vi "Set Slaves in HWI.vi"(8 "error in (no error)":errorcluster, 10 "Slave Info":T1, 11 "Pulseblaster in":refnum<class "Pulseblaster.lvclass">) -> (0 "error out":errorcluster, 3 "Pulseblaster out":refnum<class "Pulseblaster.lvclass">)   [LabVIEW 2013, in "Pulseblaster.lvclass"]
uses:
  Pulseblaster.lvclass
  TypeDefs/SlaveInfo.ctl
  TypeDefs/RampInfo.ctl
  Pulseblaster.lvclass/Pulseblaster.ctl
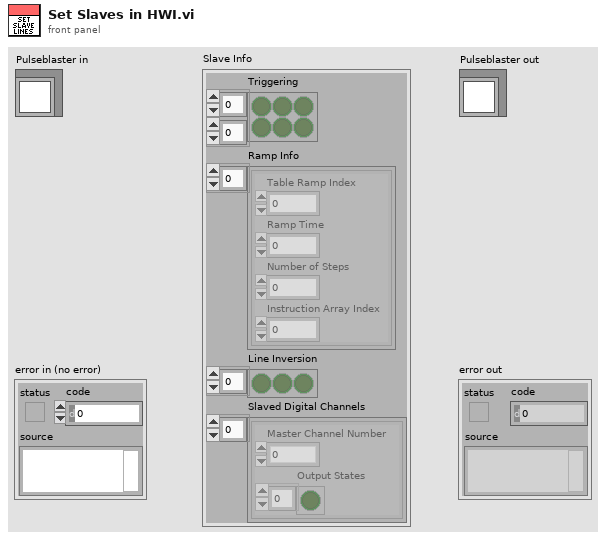
[diagram p1: front panel]
types:
  T1 = typedef "SlaveInfo.ctl" = cluster{"Triggering":bool[][], "Ramp Info":T2[], "Line Inversion":bool[], "Slaved Digital Channels":cluster{"Master Channel Number":i32, "Output States":bool[]}[]}
  T2 = typedef "RampInfo.ctl" = cluster{"Table Ramp Index":i32, "Ramp Time":dbl, "Number of Steps":i32, "Instruction Array Index":i32}
  T3 = cluster{"Master Channel Number":i32, "Output States":bool[]}[]
  T4 = cluster{"Output Bits":u32, "Data Field":u32, "OP Code":u8, "Delay Count":u64}[]
  T5 = cluster{"Output Bits":u32, "Data Field":u32, "OP Code":u8, "Delay Count":u64}
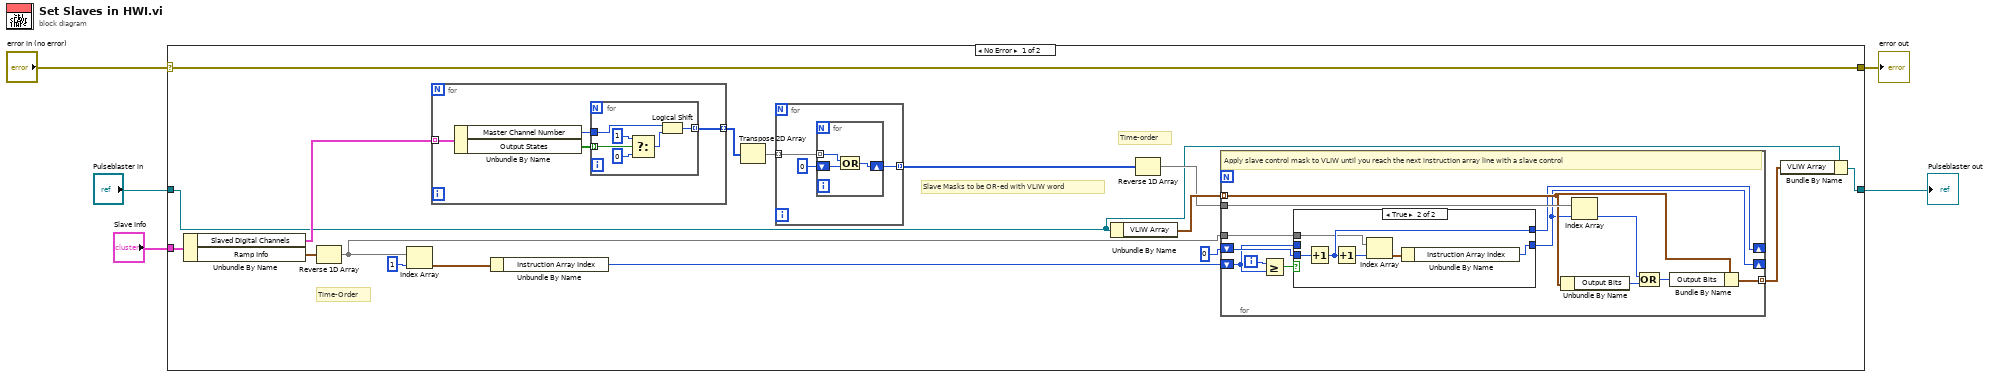
[diagram p0: block diagram]
diagram:
  n1 = case shown="No Error" "error in (no error)" {
    selector: "error in (no error)" -> [w22 w61]
    tunnel: [w22 w61] -> w4
    tunnel: [w8 w60] -> w2
    tunnel: "Pulseblaster in" -> [w6 w60]
    tunnel: "Slave Info" -> [w21 _]
    frame No Error {
      # "Slave Masks to be OR-ed with VLIW word"
      # "Time-Order"
      # "Time-order"
      n2 = Unbundle By Name(w21) -> ("Slaved Digital Channels"=w20:T3, "Ramp Info"=w15:T2[])
      n3 = Reverse 1D Array(array=w15) -> (reversed array=w11:T2[])
      n4 = Index Array(array=w11, index=1) -> (element=w13:T2)
      n5 = for {
        tunnel: w20 -> [w53] mode=indexing
        tunnel: [w50] -> w19 mode=indexing
        n6 = Unbundle By Name(w53) -> ("Master Channel Number"=w52:i32, "Output States"=w51:bool[])
        n7 = for {
          tunnel: w52 -> [w54]
          tunnel: w51 -> [w57] mode=indexing
          tunnel: [w56] -> w50 mode=indexing
          n8 = Select(t=1, s=w57, f=0) -> (s? t:f=w55:i32)
          n9 = Logical Shift(y=w54, x=w55) -> (x << y=w56:i32)
        }
      }
      n10 = Unbundle By Name(w13) -> ("Instruction Array Index"=w12:i32)
      n11 = Transpose 2D Array(2D array=w19) -> (transposed array=w18:i32[][])
      n12 = for {
        tunnel: w18 -> [w46] mode=indexing
        tunnel: [w44] -> w16 mode=indexing
        n13 = for {
          tunnel: w46 -> [w49] mode=indexing
          shift-right: [w48] -> w44
          shift-left: u32 0 ("Output Bits") -> [w47]
          n14 = Compound Arithmetic op=OR(w49, w47) -> (w48:u32)
        }
      }
      n15 = Unbundle By Name(w6) -> ("VLIW Array"=w17:T4)
      n16 = Reverse 1D Array(array=w16) -> (reversed array=w10:u32[])
      n17 = for {
        tunnel: w17 -> [w32] mode=indexing
        shift-right: [w23] -> _
        shift-left: w12 -> [w24]
        tunnel: w11 -> [w25]
        tunnel: w10 -> [w35]
        shift-right: [w26] -> _
        shift-left: 0 ("index") -> [w27]
        tunnel: [w30] -> w7 mode=indexing
        i -> [w29]
        # "Apply slave control mask to VLIW until you reach the next instruction array line with a slave control"
        n18 = Greater Or Equal?(x=w29, y=w24) -> (x >= y?=w28:bool)
        n19 = case shown="True" w28 {
          tunnel: w27 -> [w37 w43]
          tunnel: [w37 w42] -> w26
          tunnel: w25 -> [_ w40]
          tunnel: [w36 w38] -> w23
          tunnel: w24 -> [w36 _]
          frame False {
          }
          frame True {
            n20 = Increment(x=w43) -> (x+1=w42:i32)
            n21 = Increment(x=w42) -> (x+1=w41:i32)
            n22 = Index Array(array=w40, index=w41) -> (element=w39:T2)
            n23 = Unbundle By Name(w39) -> ("Instruction Array Index"=w38:i32)
          }
        }
        n24 = Unbundle By Name(w32) -> ("Output Bits"=w33:u32)
        n25 = Index Array(array=w35, index=w23) -> (element=w34:u32)
        n26 = Compound Arithmetic op=OR(w34, w33) -> (w31:u32)
        n27 = Bundle By Name(cluster=w32, "Output Bits"=w31) -> (w30:T5)
      }
      n28 = Bundle By Name(cluster=w6, "VLIW Array"=w7) -> (w8:refnum<class "Pulseblaster.lvclass">)
    }
    frame Error {
    }
  }
  "error out" <- w4
  "Pulseblaster out" <- w2
